vi "Instrument.1820.FloatApprox.vi"(4 "y":dbl, 5 "x":dbl) -> (1 "x ~ y?":bool)   [LabVIEW 2016, in "Instrument.OxfordVRM.lvclass"]
doc: "Use to compare floating point numbers. This will check if two numbers are the same to 6 decimal places. Edit block diagram to change tolerance."
uses:
  Instrument.OxfordVRM.lvclass
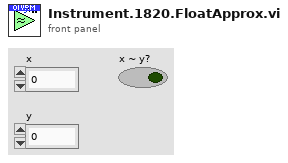
[diagram p1: front panel]
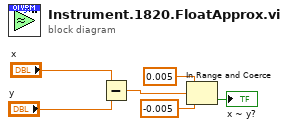
[diagram p0: block diagram]
diagram:
  n1 = Subtract(x="x", y="y") -> (x-y=w3:dbl)
  n2 = In Range and Coerce(upper limit=0.005, x=w3, lower limit=-0.005 ("upper limit")) -> (In Range?=→"x ~ y?":bool)  [unwired: 1 out]
